vi "AudioTest.SoundCheck Data Log Analysis_Module.vi"(6 "PlotColors":u32[](array[colorbox])=[56063, 16776722, 16730898, 16711925, 6618880], 7 "LimColors":u32[](array[colorbox])=[16448250, 16448250, 16448250, 16448250, 16448250, 16448250], 11 "Module Config":T3={"Name"="AudioGraphs", "Parent Q"=refnum, "Is Child?"=FALSE, "Index"=0, "Dirs"={"Root"=path "", "Config"=path "C:/MTE/Audio Test/Config", "Logs"=path "", "Reports"=path "", "App Data"=path ""}, "Simulate"=FALSE, "SimCtrl"=refnum}) -> ()   [LabVIEW 2018]
uses:
  <vilib>/KATE/Module/Module Config.ctl
  <vilib>/KATE/Queues/Q.Element.ctl
  <vilib>/KATE/Module/Module.Working Dirs.ctl
  Common/Utils/Results/Result.Measurement Item.ctl
  Common/Utils/Results/Result.Measurement and Attribute Item Status.ctl
  TypeDefs/AudioTest.Analysis Data Record.ctl
  TypeDefs/AudioTest.Analysis Folder Navigation Status.ctl
  Common/Utils/Errors/Error.Error Code List.ctl
  <vilib>/KATE/Queues/Queue Utils.lvlib
  <vilib>/KATE/Files/File Utils.lvlib
  <vilib>/KATE/Time/Time Utils.lvlib
  <vilib>/KATE/Module/Module Utils.lvlib
panel:
  in  "Main Tab":enum32{"Graphs", "Results", "Setup"}(tab)
  in  "Graph - Open Composite Sm":bool
  in  "UUT Dir Order":enum16{"Name", "Date"}(ring)
  in  "UUTDir Next":bool
  in  "UUTDir Prev":bool
  in  "Graph - Open Composite":bool
  in  "Go To Results":bool
  in  "Graph Wins - Reset Pos":bool
  in  "Graph Wins - Close":bool
  in  "Graph Wins - Open":bool
  in  "Save to CSV":bool
  in  "X Scale":enum16{"Log", "Linear"}(ring)
  out "Y Units":string
  out "X Units":string
  in  "Next":bool
  in  "Prev":bool
  out "XY Graph":cluster{"X":dbl[], "Y":dbl[]}[](graph)
  in  "Plot":u16(ring)
  in  "SoundCheck Data File":path caption="Data File"
  in  "Load File":bool
  in  "Go To Setup":bool
  in  "Go To Graphs":bool
  out "Meas Data":T1[](array[typedef]) {"Status" items=["LOG", "PASS", "FAIL", "ERROR"]}
  in  "Reinit Config":bool
  out "Graph Cnt":i32
  out "Error":errorcluster
  out "Q Name":string="AudioGraphs"
  in  "Go To Graphs 2":bool
  # "Indiv Graphs"
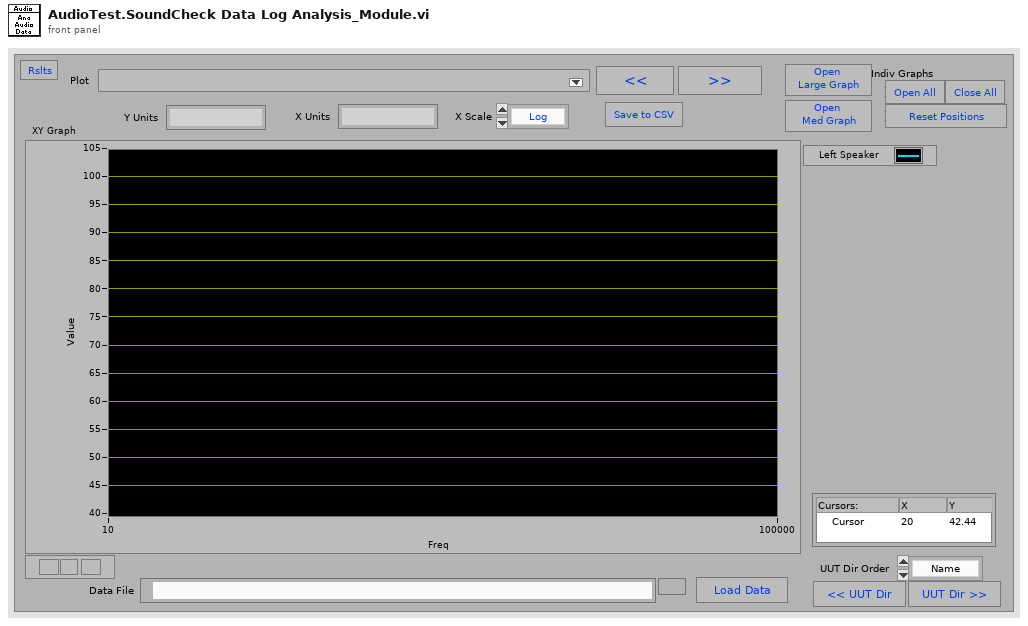
[diagram p1: front panel]
types:
  T1 = typedef "Result.Measurement Item.ctl" = cluster{"Cnt":i32, "Step":string, "Category":string, "Name":string, "Value":string, "Units":string, "LimType":string, "LL":string, "UL":string, "Status":T2, "Code":i32, "Desc":string, "Time":timestamp}
  T2 = typedef "Result.Measurement and Attribute Item Status.ctl" = i32
  T3 = typedef "KATE_Lib.lvlib/Module Utils.lvlib/Module Config.ctl" = cluster{"Name":string, "Parent Q":refnum<queue>, "Is Child?":bool, "Index":i32, "Dirs":T4, "Simulate":bool, "SimCtrl":refnum<vi>}
  T4 = typedef "KATE_Lib.lvlib/Module Utils.lvlib/Module.Working Dirs.ctl" = cluster{"Root":path, "Config":path, "Logs":path, "Reports":path, "App Data":path}
  T5 = typedef "AudioTest.Analysis Data Record.ctl" = cluster{"Name":string, "X Units":string, "Y Units":string, "DataPlots":cluster{"X":dbl[], "Y":dbl[]}[], "LimitPlots":cluster{"X":dbl[], "Y":dbl[]}[], "DataPlotNames":string[], "LimitPlotNames":string[], "Fail":bool}
  T6 = typedef "AudioTest.Analysis Folder Navigation Status.ctl" = cluster{"Index":i32, "Count":i32, "HightEnd":bool, "LowtEnd":bool}
  T7 = enum32{"invalid app kind", "Development System", "Run Time System", "Student Edition", "Embedded LabVIEW", "Evaluation", "Custom"}
  T8 = cluster{"Graphs":T5[], "Config Dir":path, "PlotColors":u32[], "LimColors":u32[], "PlotWins":cluster{"Name":string, "vi ref":refnum<vi>}[], "PlotComp":cluster{"Name":string, "vi ref":refnum<vi>}, "DataFolder":path, "DirNavStatus":T6}
  T9 = typedef "Error.Error Code List.ctl" = i32
  T10 = typedef "KATE_Lib.lvlib/Queue Utils.lvlib/Q.Element.ctl" = cluster{"Cmd":string, "Sub":string, "Data1":variant, "Data2":variant}
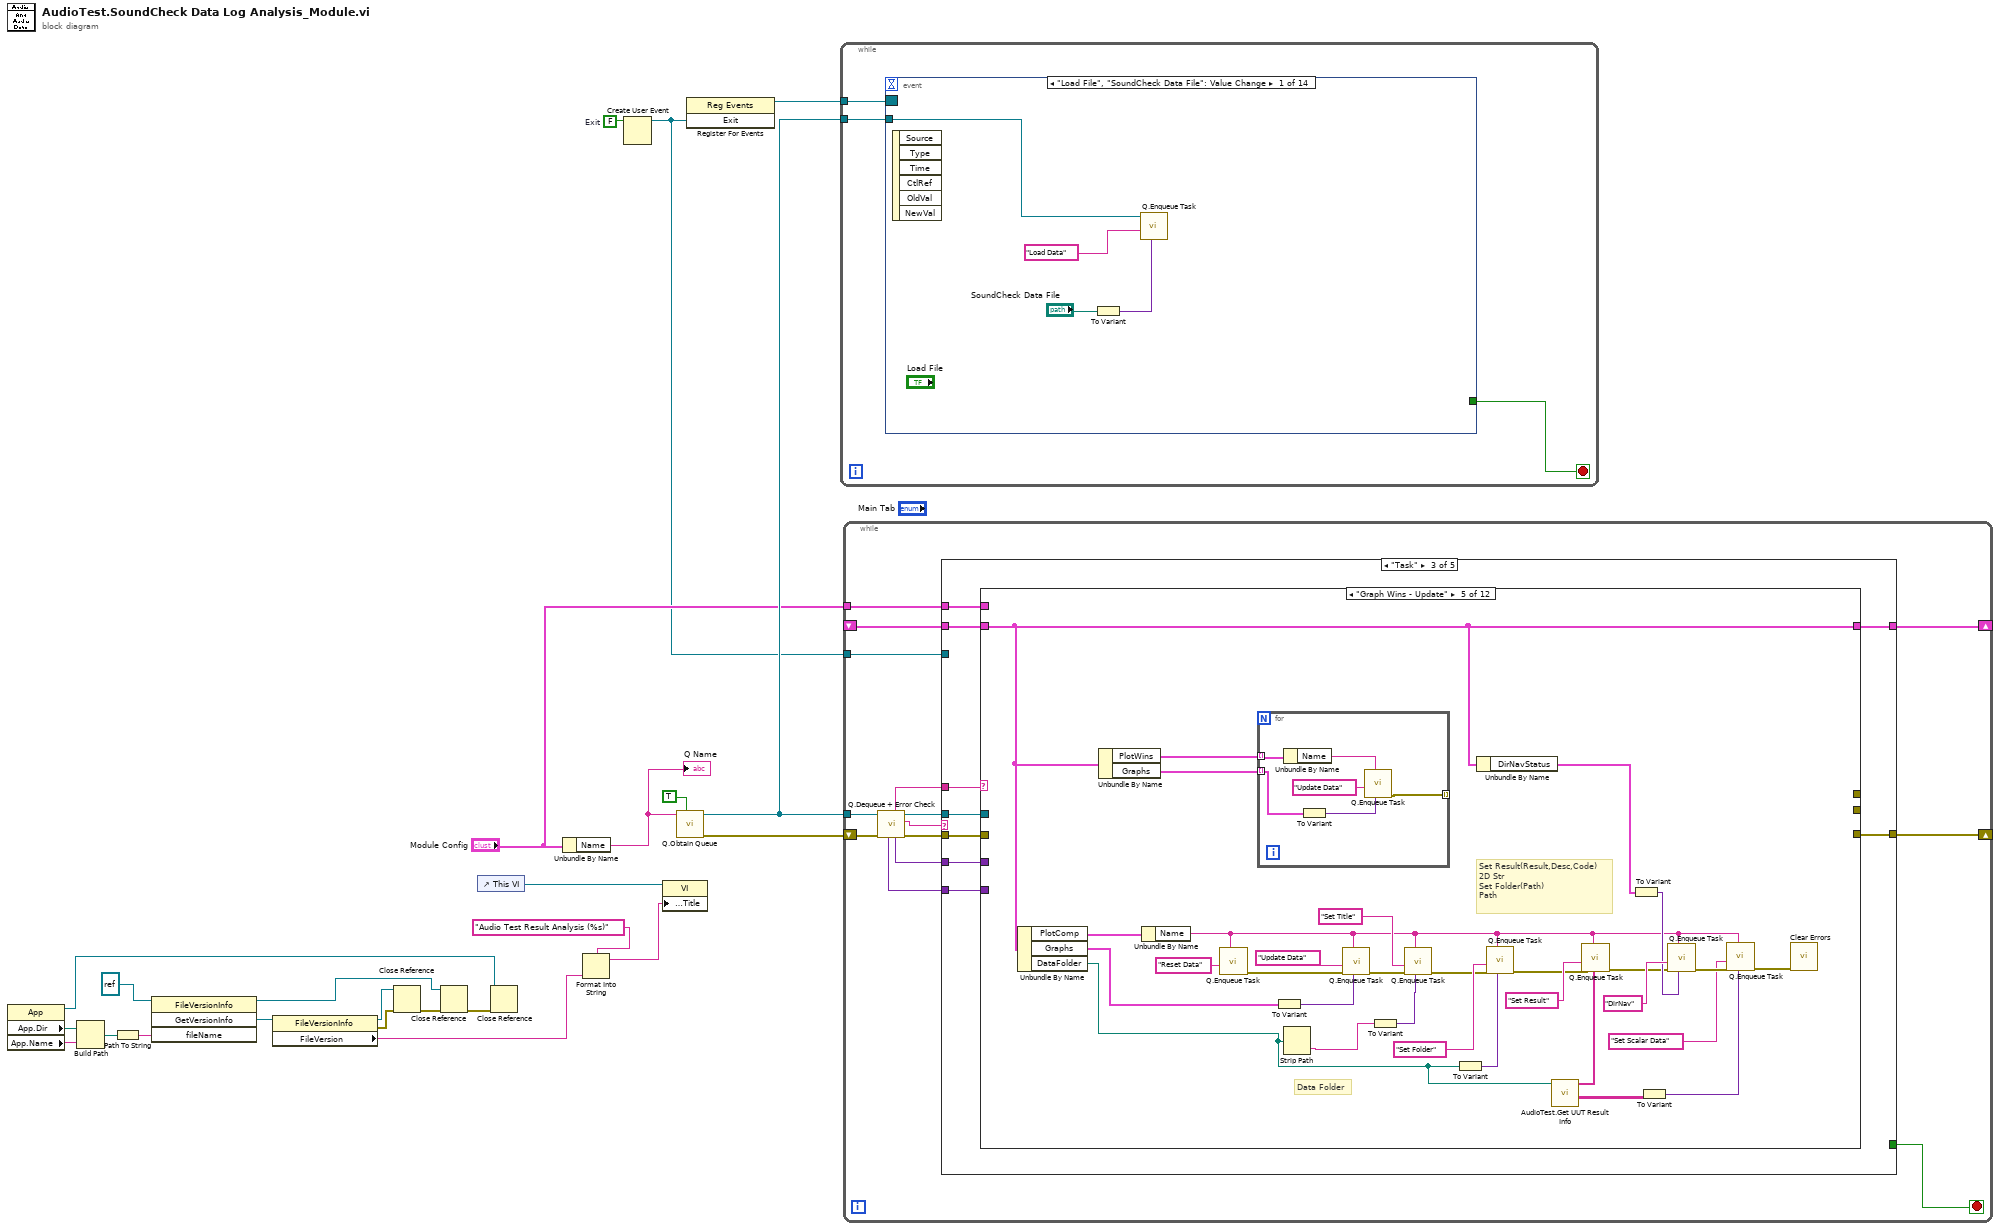
[diagram p0: block diagram]
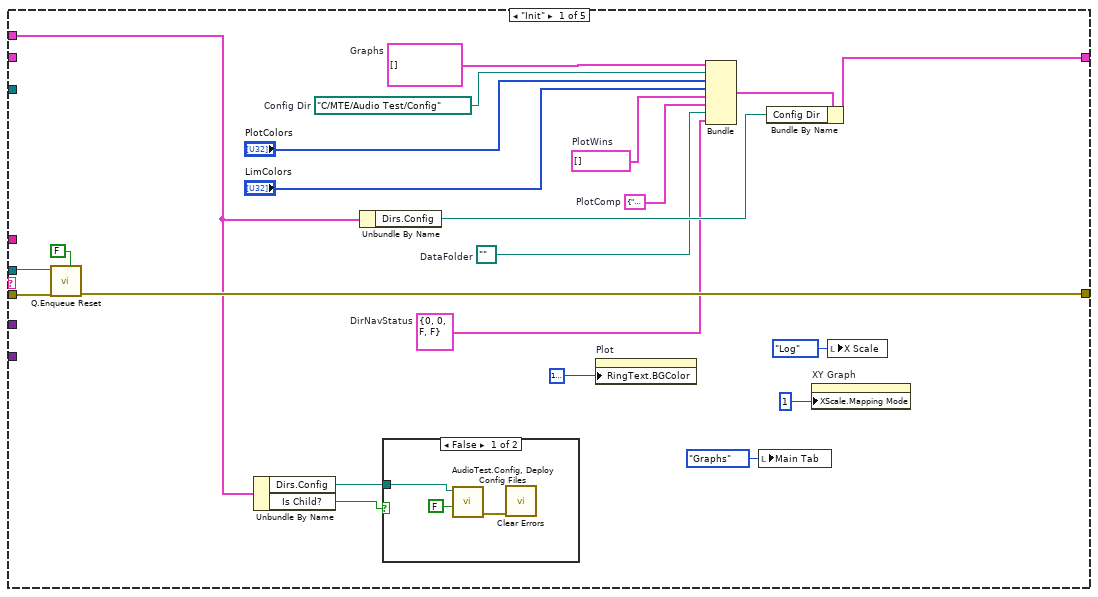
[diagram p2: hidden frame]
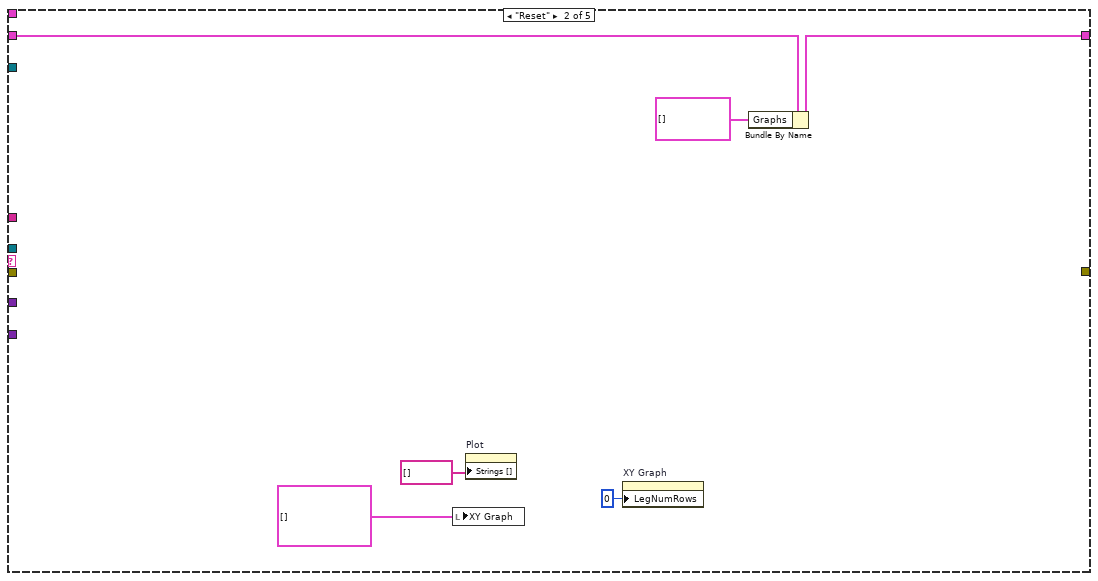
[diagram p4: hidden frame]
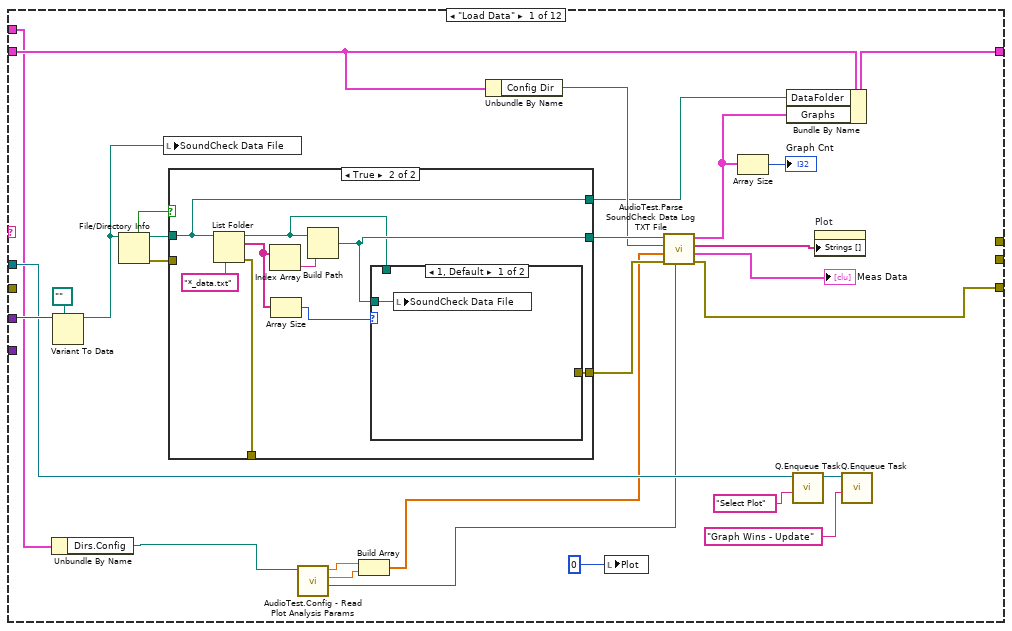
[diagram p5: hidden frame]
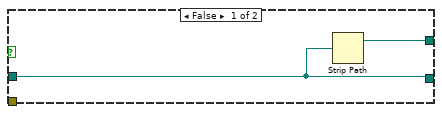
[diagram p6: hidden frame]
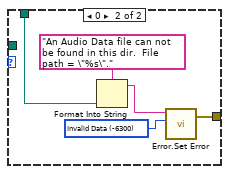
[diagram p7: hidden frame]
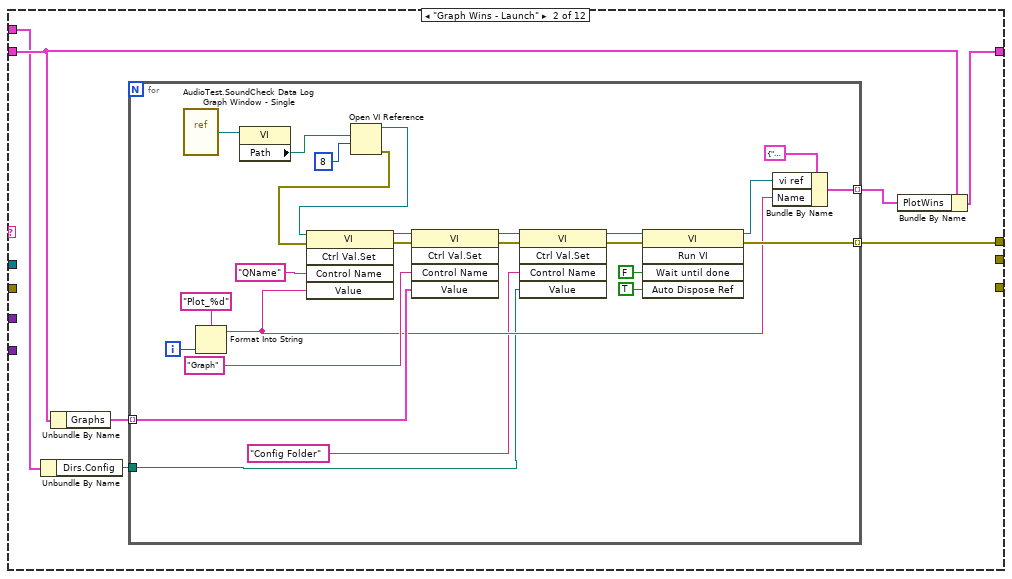
[diagram p8: hidden frame]
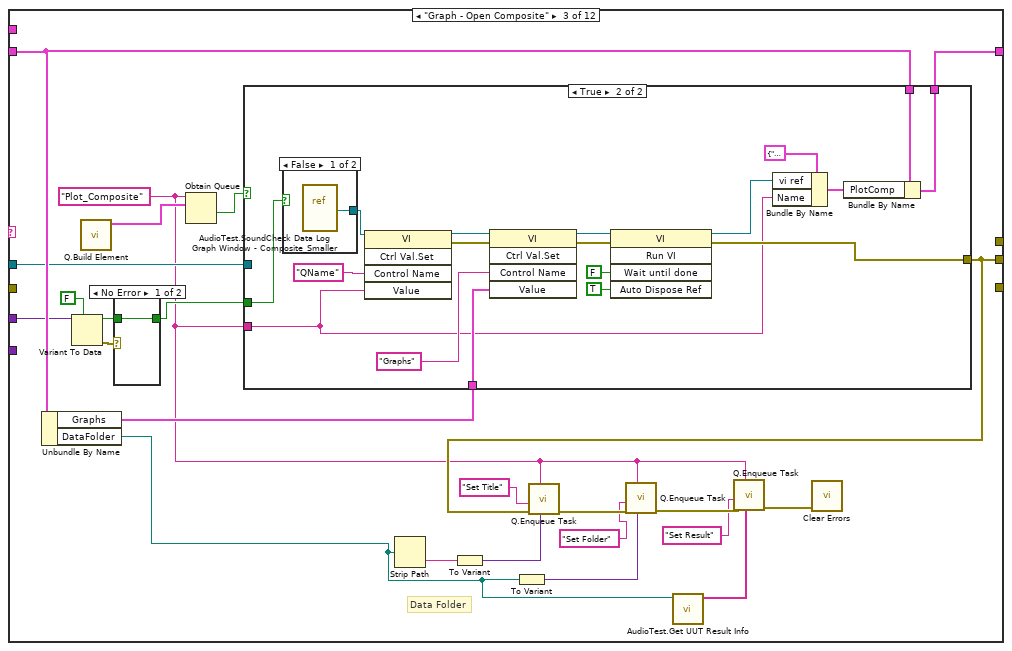
[diagram p9: hidden frame]
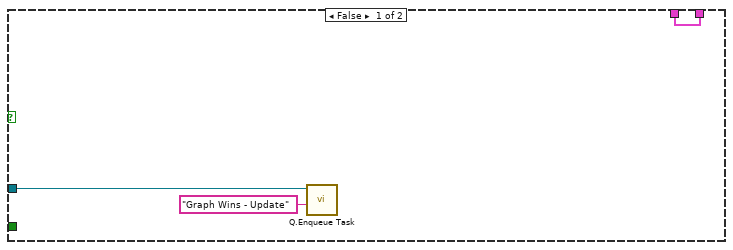
[diagram p11: hidden frame]
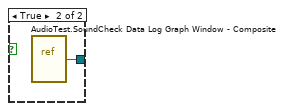
[diagram p12: hidden frame]
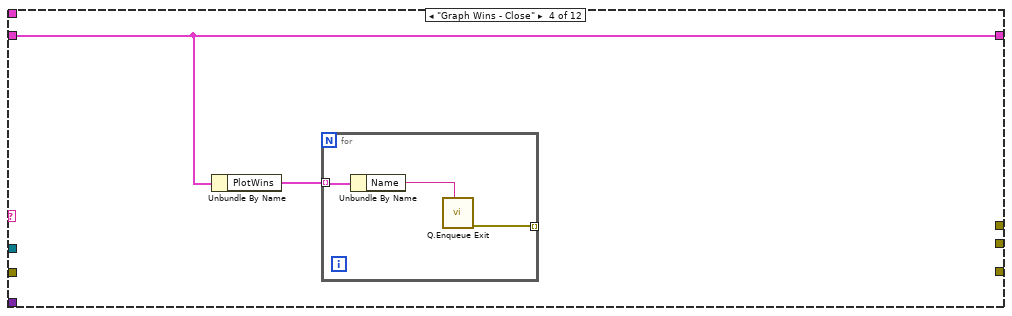
[diagram p13: hidden frame]
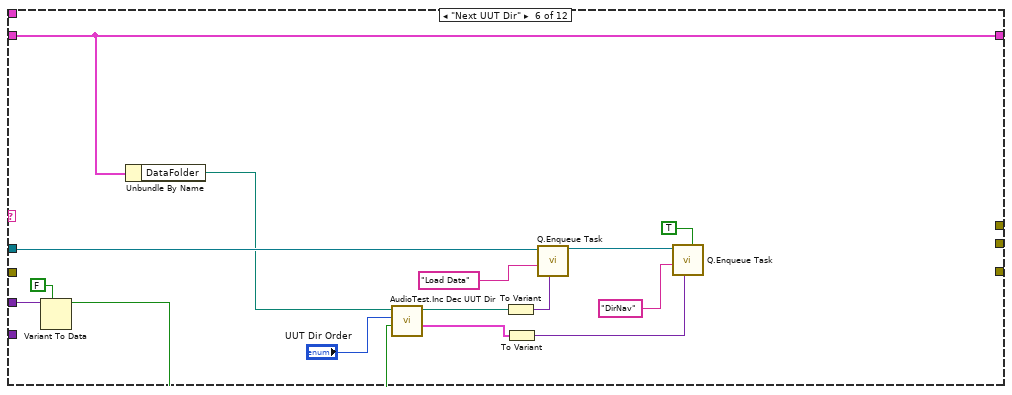
[diagram p14: hidden frame]
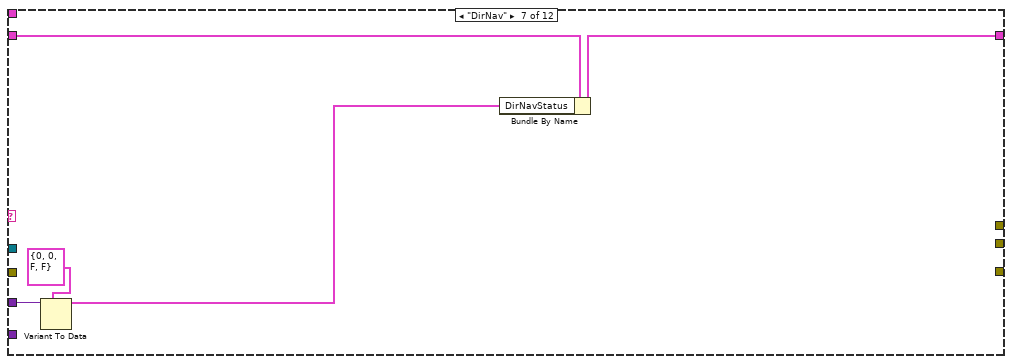
[diagram p15: hidden frame]
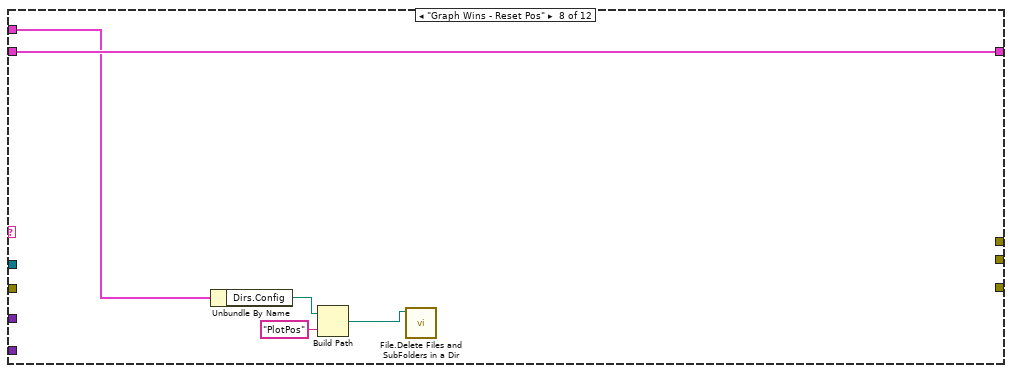
[diagram p16: hidden frame]
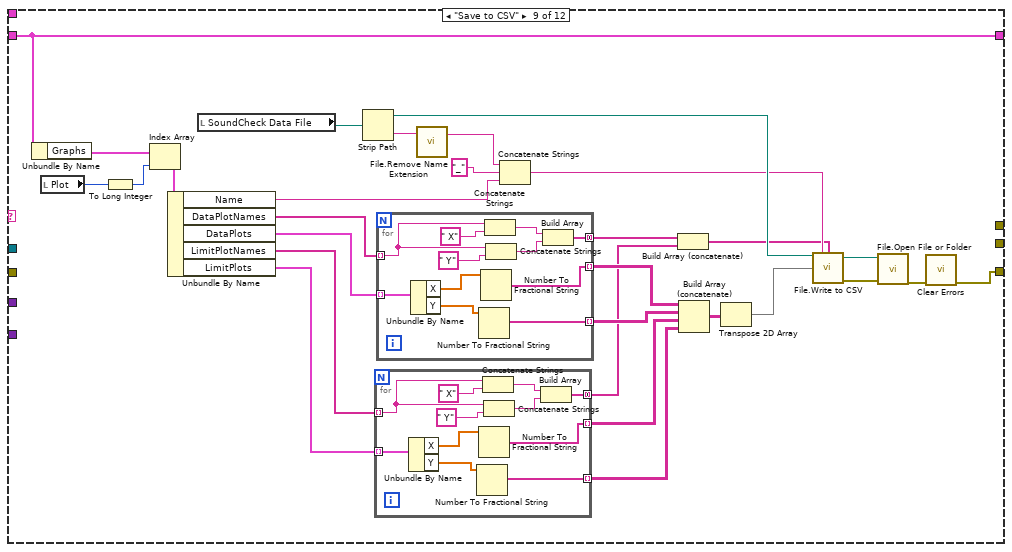
[diagram p17: hidden frame]
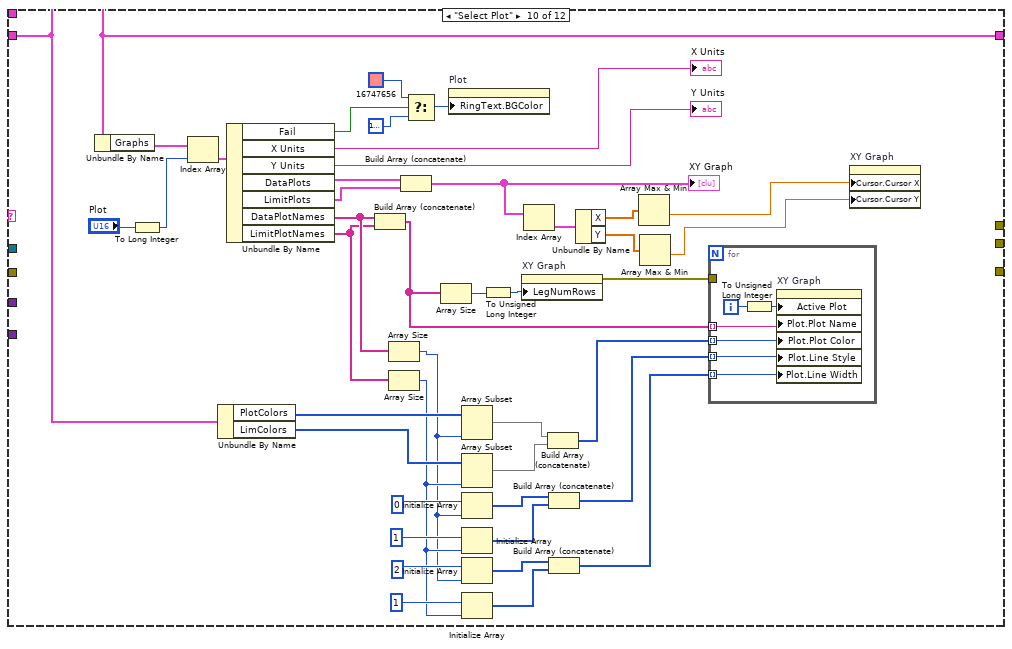
[diagram p18: hidden frame]
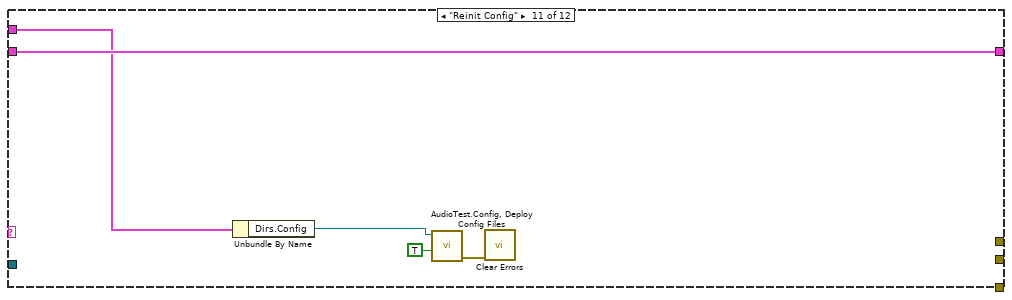
[diagram p19: hidden frame]
diagram:
  w24 = FALSE  # Exit
  n1 = property class="App"() -> (reference out=w3:refnum<vi>, "App.Dir"=w7:path, "App.Name"=w6:string)  [unwired: 2 in, 1 out]
  n2 = Build Path(base path=w7, name or relative path=w6) -> (appended path=w5:path)
  n3 = Path To String(path=w5) -> (string=w13:string)
  n4 = invoke class="FileVersionInfo" method="GetVersionInfo"(reference=refnum<k24> refnum, "fileName"=w13) -> (reference out=w9:refnum<k24>, "GetVersionInfo"=w14:refnum<k24>)  [unwired: 2 in, 2 out]
  n5 = property class="FileVersionInfo"(reference=w14) -> (reference out=w12:refnum<k24>, error out=w11:errorcluster, "FileVersion"=w2:string)  [unwired: 1 in]
  n6 = Close Reference(reference=w12, error in (no error)=w11) -> (error out=w10:errorcluster)
  n7 = Close Reference(reference=w9, error in (no error)=w10) -> (error out=w4:errorcluster)
  n8 = control-ref of="This VI"() -> (w17:refnum<vi>)
  n9 = Close Reference(reference=w3, error in (no error)=w4) -> ()  [unwired: 1 out]
  n10 = Unbundle By Name("Module Config") -> ("Name"=w19:string)
  "Q Name" <- w19
  n11 = Format Into String(format string="Audio Test Result Analysis (%s)", w2) -> (resulting string=w15:string)  [unwired: 2 in, 1 out]
  n12 = Create User Event(user event datatype=w24) -> (user event=w1:refnum<user-event>)  [unwired: 1 in, 1 out]
  n13 = property class="VI"(reference=w17, "Front Panel.Title"=w15) -> ()  [unwired: 1 in, 2 out]
  n14 = call <vilib>:"Q.Obtain Queue.vi"("Enqueue Init"=TRUE, "Q Name"=w19) -> ("error out"=w21:errorcluster, "Q Out"=w20:refnum<queue>)  [unwired: 7 in, 1 out]
  n15 = register-events(w1) -> (reference out=w23:refnum<event-registration>)  [unwired: 2 in, 1 out]
  n16 = while {
    tunnel: w23 -> [w27]
    tunnel: w20 -> [w26]
    stop <- w25 stop-if-true
    n17 = event shown="[0] \"Load File\", \"SoundCheck Data File\": Value Change" {
      selector: w27 -> [_ _ _ _ _ _ _ _ _ _ _ _ _ _]
      dyn-events: _ -> [_ _ _ _ _ _ _ _ _ _ _ _ _ _]
      timeout: _ -> [_ _ _ _ _ _ _ _ _ _ _ _ _ _]
      tunnel: w26 -> [w30 w33 _ w46 w48 w50 w53 w59 w60 w62 _ w75 w89 w92]
      tunnel: [_ _ _ _ _ _ _ _ _ _ _ _ w90 TRUE] -> w25
      event "Load File", "SoundCheck Data File": Value Change {
        n18 = event-data() -> ()  [unwired: 1 in, 6 out]
        n19 = To Variant(anything="SoundCheck Data File") -> (Variant=w28:variant)
        n20 = call <vilib>:"Q.Enqueue Task.vi"("Data1"=w28, "Task Name"="Load Data", "Q In"=w30) -> ()  [unwired: 7 in, 2 out]
      }
      event "UUTDir Prev", "UUTDir Next": Value Change {
        n21 = event-data() -> ()  [unwired: 1 in, 6 out]
        n22 = To Variant(anything="UUTDir Next") -> (Variant=w34:variant)
        n23 = call <vilib>:"Q.Enqueue Task.vi"("Data1"=w34, "Task Name"="Next UUT Dir", "Q In"=w33) -> ()  [unwired: 7 in, 2 out]
      }
      event "Go To Setup", "Go To Results", "Go To Graphs 2", "Go To Graphs": Value Change {
        n24 = event-data() -> ()  [unwired: 1 in, 6 out]
        n25 = Or(x="Go To Graphs 2", y="Go To Graphs") -> (x .or. y?=w37:bool)
        n26 = case shown="False" w37 {
          tunnel: [w42 enum32{"Graphs", "Results", "Setup"}."Graphs" ("Main Tab")] -> w40
          tunnel: "Go To Results" -> [w41 _]
          frame False {
            n27 = case shown="False" w41 {
              tunnel: [enum32{"Graphs", "Results", "Setup"}."Setup" ("Main Tab") enum32{"Graphs", "Results", "Setup"}."Results" ("Main Tab")] -> w42
              frame False {
              }
              frame True {
              }
            }
          }
          frame True {
          }
        }
        n28 = local write "Main Tab"(w40) -> ()
      }
      event "Reinit Config": Value Change {
        n29 = event-data() -> ()  [unwired: 1 in, 6 out]
        n30 = call <vilib>:"Q.Enqueue Task.vi"("Task Name"="Reinit Config", "Q In"=w46) -> ()  [unwired: 8 in, 2 out]
      }
      event "Plot": Value Change {
        n31 = event-data() -> ()  [unwired: 1 in, 6 out]
        n32 = call <vilib>:"Q.Enqueue Task.vi"("Task Name"="Select Plot", "Q In"=w48) -> ()  [unwired: 8 in, 2 out]
      }
      event "Save to CSV": Value Change {
        n33 = event-data() -> ()  [unwired: 1 in, 6 out]
        n34 = call <vilib>:"Q.Enqueue Task.vi"("Task Name"="Save to CSV", "Q In"=w50) -> ()  [unwired: 8 in, 2 out]
      }
      event "Graph Wins - Open": Value Change {
        n35 = event-data() -> ()  [unwired: 1 in, 6 out]
        n36 = call <vilib>:"Q.Enqueue Task.vi"("Task Name"="Graph Wins - Close", "Q In"=w53) -> ("Q Out"=w52:refnum<queue>)  [unwired: 8 in, 1 out]
        n37 = call <vilib>:"Q.Enqueue Task.vi"("Task Name"="Graph Wins - Launch", "Q In"=w52) -> ()  [unwired: 8 in, 2 out]
      }
      event "Graph - Open Composite", "Graph - Open Composite Sm": Value Change {
        n38 = event-data() -> ()  [unwired: 1 in, 6 out]
        n39 = To Variant(anything="Graph - Open Composite") -> (Variant=w57:variant)
        n40 = call <vilib>:"Q.Enqueue Task.vi"("Data1"=w57, "Task Name"="Graph - Open Composite", "Q In"=w59) -> ()  [unwired: 7 in, 2 out]
      }
      event "Graph Wins - Reset Pos": Value Change {
        n41 = event-data() -> ()  [unwired: 1 in, 6 out]
        n42 = call <vilib>:"Q.Enqueue Task.vi"("Task Name"="Graph Wins - Reset Pos", "Q In"=w60) -> ()  [unwired: 8 in, 2 out]
      }
      event "Graph Wins - Close": Value Change {
        n43 = event-data() -> ()  [unwired: 1 in, 6 out]
        n44 = call <vilib>:"Q.Enqueue Task.vi"("Task Name"="Graph Wins - Close", "Q In"=w62) -> ()  [unwired: 8 in, 2 out]
      }
      event "X Scale": Value Change {
        n45 = event-data() -> ()  [unwired: 1 in, 6 out]
        n46 = case shown="\"Log\", Default" "X Scale" {
          tunnel: [u8 1 u8 0] -> w64
          frame "Log", Default {
          }
          frame "Linear" {
          }
        }
        n47 = property on="XY Graph" class="XYGraph (strict)"("XScale.Mapping Mode"=w64) -> ()  [unwired: 2 in, 2 out]
      }
      event "Next", "Prev": Value Change {
        n48 = event-data() -> ()  [unwired: 1 in, 6 out]
        n49 = local read "Graph Cnt"() -> (w71:i32)
        n50 = local read "Plot"() -> (w73:u16)
        n51 = Decrement(x=w71) -> (x-1=w70:i32)
        n52 = To Long Integer(number=w73) -> (32bit integer=w72:i32)
        n53 = case shown="False" "Next" {
          tunnel: w72 -> [w81 w87]
          tunnel: [w77 w85] -> w69
          tunnel: w70 -> [w80 w86]
          frame False {
            n54 = Decrement(x=w81) -> (x-1=w78:i32)
            n55 = Less Than 0?(x=w78) -> (x < 0?=w79:bool)
            n56 = Select(t=w80, s=w79, f=w78) -> (s? t:f=w77:i32)
          }
          frame True {
            n57 = Increment(x=w87) -> (x+1=w82:i32)
            n58 = Greater?(x=w82, y=w86) -> (0:w84:bool)
            n59 = Select(t=0, s=w84, f=w82) -> (s? t:f=w85:i32)
          }
        }
        n60 = To Unsigned Word Integer(number=w69) -> (unsigned 16bit integer=w68:u16)
        n61 = call <vilib>:"Q.Enqueue Task.vi"("Task Name"="Select Plot", "Q In"=w75) -> ()  [unwired: 8 in, 2 out]
        n62 = local write "Plot"(w68) -> ()
      }
      event Panel Close? {
        w90 = TRUE
        n63 = event-data() -> ()  [unwired: 1 in, 4 out]
        n64 = call <vilib>:"Q.Enqueue Exit.vi"("Q In"=w89) -> ("error out"=w88:errorcluster)  [unwired: 9 in, 1 out]
        n65 = call <vilib>:"Clear Errors.vi"("error in (no error)"=w88) -> ()  [unwired: 5 in, 2 out]
        n66 = event-data("Discard?"=w90) -> ()  [unwired: 1 in, 1 out]
      }
      event User Event {
        n67 = event-data() -> ()  [unwired: 1 in, 5 out]
        n68 = call <vilib>:"Q.Enqueue Exit.vi"("Q In"=w92) -> ("error out"=w91:errorcluster)  [unwired: 9 in, 1 out]
        n69 = call <vilib>:"Clear Errors.vi"("error in (no error)"=w91) -> ()  [unwired: 5 in, 2 out]
      }
    }
  }
  n70 = while {
    shift-right: [w99] -> _
    shift-left: w21 -> [w104]
    tunnel: w20 -> [w102]
    shift-right: [w97] -> _
    shift-left: _ -> [w96]
    tunnel: "Module Config" -> [w95]
    tunnel: w1 -> [w94]
    stop <- w98 stop-if-true
    n71 = call <vilib>:"Q.Dequeue + Error Check.vi"("Error In"=w104, "Q In"=w102) -> ("error out"=w105:errorcluster, "Cmd"=w107:string, "Q Out"=w106:refnum<queue>, "Data1"=w101:variant, "Sub"=w103:string, "Data2"=w100:variant)  [unwired: 4 in]
    n72 = case shown="\"Task\"" w107 {
      tunnel: w106 -> [w129 _ w146 w446 _]
      tunnel: w105 -> [w128 _ w145 w445 _]
      tunnel: w103 -> [_ _ w147 _ _]
      tunnel: w101 -> [_ _ w144 _ _]
      tunnel: w100 -> [_ _ w143 _ _]
      tunnel: [w126 _ w140 _ _] -> w99
      tunnel: [_ _ _ _ TRUE] -> w98
      tunnel: [w118 w137 w141 w448 w458] -> w97
      tunnel: w96 -> [_ w136 w142 w448 w458]
      tunnel: w95 -> [w111 _ w139 _ w462]
      tunnel: w94 -> [_ _ _ _ w450]
      frame "Init" {
        w108 = T6 {"Index"=0, "Count"=0, "HightEnd"=FALSE, "LowtEnd"=FALSE}  # DirNavStatus
        w109 = path ""  # DataFolder
        w114 = cluster{"Name":string, "vi ref":refnum<vi>} {"Name"="", "vi ref"=refnum}  # PlotComp
        w116 = cluster{"Name":string, "vi ref":refnum<vi>}[] []  # PlotWins
        w122 = path "C:/MTE/Audio Test/Config"  # Config Dir
        w125 = T5[] []  # Graphs
        n73 = call <vilib>:"Q.Enqueue Reset.vi"("Top of Q(T)"=FALSE, "Error In"=w128, "Q In"=w129) -> ("error out"=w126:errorcluster)  [unwired: 7 in, 1 out]
        n74 = Unbundle By Name(w111) -> ("Dirs.Config"=w112:path, "Is Child?"=w110:bool)
        n75 = Unbundle By Name(w111) -> ("Dirs.Config"=w117:path)
        n76 = case shown="False" w110 {
          tunnel: w112 -> [w131 _]
          frame False {
            n77 = call "AudioTest.Config, Deploy Config Files.vi"("SkipIfExists(F)/Overwrite(T)"=FALSE, "Config Folder"=w131) -> ("error out"=w132:errorcluster)  [unwired: 9 in]
            n78 = call <vilib>:"Clear Errors.vi"("error in (no error)"=w132) -> ()  [unwired: 5 in, 2 out]
          }
          frame True {
          }
        }
        n79 = property on="Plot" class="Ring (strict)"("RingText.BGColor"=u32 16777216 ("Color Box")) -> ()  [unwired: 2 in, 2 out]
        n80 = Bundle("Graphs"=w125, "Config Dir"=w122, "PlotColors"="PlotColors", "LimColors"="LimColors", "PlotWins"=w116, "PlotComp"=w114, "DataFolder"=w109, "DirNavStatus"=w108) -> (w119:T8)  [unwired: 1 in]
        n81 = local write "Main Tab"(enum32{"Graphs", "Results", "Setup"}."Graphs" ("Main Tab")) -> ()
        n82 = Bundle By Name(cluster=w119, "Config Dir"=w117) -> (w118:T8)
        n83 = property on="XY Graph" class="XYGraph (strict)"("XScale.Mapping Mode"=u8 1) -> ()  [unwired: 2 in, 2 out]
        n84 = local write "X Scale"(enum16{"Log", "Linear"}."Log" ("X Scale")) -> ()
      }
      frame "Reset" {
        n85 = local write "XY Graph"(cluster{"X":dbl[], "Y":dbl[]}[] [] ("appended array")) -> ()
        n86 = property on="Plot" class="Ring (strict)"("Strings []"=string[] []) -> ()  [unwired: 2 in, 2 out]
        n87 = property on="XY Graph" class="XYGraph (strict)"("LegNumRows"=u32 0 ("Legend:Number of Rows")) -> ()  [unwired: 2 in, 2 out]
        n88 = Bundle By Name(cluster=w136, "Graphs"=T5[] []) -> (w137:T8)
      }
      frame "Task" {
        n89 = case shown="\"Graph Wins - Update\"" w147 {
          tunnel: w146 -> [w166 _ w238 _ _ w324 _ _ _ _ _ _]
          tunnel: w145 -> [_ _ _ _ _ _ _ _ _ _ _ _]
          tunnel: w144 -> [w169 _ w243 _ _ w323 w333 _ _ _ _ _]
          tunnel: w143 -> [_ _ _ _ _ _ _ _ _ _ _ _]
          tunnel: w142 -> [w162 w198 w246 w274 w286 w320 w330 w338 w363 w419 w442 w443]
          tunnel: [w167 w197 w245 w274 w286 w320 w331 w338 w363 w419 w442 w443] -> w141
          tunnel: [w165 _ _ _ _ _ _ _ w340 _ _ _] -> w140
          tunnel: [_ w195 _ _ _ _ _ _ _ _ _ _] -> _
          tunnel: w139 -> [w155 w194 _ _ _ _ _ w337 _ _ w440 _]
          tunnel: [_ _ w227 _ _ _ _ _ _ _ _ _] -> _
          frame "Load Data" {
            n90 = Unbundle By Name(w155) -> ("Dirs.Config"=w154:path)
            n91 = Variant To Data(type=path "", Variant=w169) -> (data=w164:path)  [unwired: 1 in, 1 out]
            n92 = File/Directory Info(path=w164) -> (path out=w171:path, directory=w172:bool, error out=w174:errorcluster)  [unwired: 1 in, 4 out]
            n93 = local write "SoundCheck Data File"(w164) -> ()
            n94 = case shown="True" w172 {
              tunnel: w171 -> [w177 w178]
              tunnel: [w177 w185] -> w173
              tunnel: w174 -> [_ _]
              tunnel: [_ w184] -> _
              tunnel: [_ w180] -> w175
              tunnel: [w176 w178] -> w148
              frame False {
                n95 = Strip Path(path=w177) -> (stripped path=w176:path)  [unwired: 1 out]
              }
              frame True {
                n96 = List Folder(path=w178, pattern="*_data.txt") -> (path out=w179:path, filenames=w183:string[], error out=w184:errorcluster)  [unwired: 2 in, 1 out]
                n97 = Index Array(array=w183) -> (element=w181:string)  [unwired: 1 in]
                n98 = Array Size(array=w183) -> (size(s)=w182:i32)
                n99 = Build Path(base path=w179, name or relative path=w181) -> (appended path=w185:path)
                n100 = case shown="1, Default" w182 {
                  tunnel: w185 -> [w187 _]
                  tunnel: [_ w189] -> w180
                  tunnel: w179 -> [_ w188]
                  frame 1, Default {
                    n101 = local write "SoundCheck Data File"(w187) -> ()
                  }
                  frame 0 {
                    w190 = T9 -6300 items=["No Error"=0, "Abort"=-2, "Misc"=-5000, "Fixture Error"=-5100, "File IO - General"=-5200, "FIle IO - Config Error"=-5201, "Instrument - General"=-5300, "Instrument - Serial Com"=-5301, "Instrument - Camera"=-5302, "Instrument - PS"=-5303, "Instrument - Oscilloscope"=-5304, "Instrument - Function Gen"=-5305, "Instrument - Load"=-5306, "Instrument - Meter"=-5307, "Instrument - Power Control"=-5308, "Instrument - Motion"=-5309, "Instrument - RF"=-5310, "System Exe"=-5400, "Image Processing"=-5500, "Communication"=-5600, "Script - Syntax Error"=-6000, "Script - Invalid Name or Param"=-6100, "Script - Timeout"=-6200, "Invalid Data"=-6300, "FW Update Error"=-6500] ("Std Code")
                    n102 = Format Into String(format string="An Audio Data file can not be found in this dir.  File path = \"%s\"." ("Desc"), w188) -> (resulting string=w192:string)  [unwired: 2 in, 1 out]
                    n103 = call "Error.Set Error.vi"("Code"=w190, "Desc"=w192) -> ("error out"=w189:errorcluster)  [unwired: 5 in]
                  }
                }
              }
            }
            n104 = call "AudioTest.Config - Read Plot Analysis Params.vi"("Config Dir"=w154) -> ("Avg(F)/Float(T)"=w152:bool, "End Freq"=w156:dbl, "Start Freq"=w157:dbl)  [unwired: 8 in]
            n105 = Build Array(w157, w156) -> (w153:dbl[])
            n106 = Unbundle By Name(w162) -> ("Config Dir"=w161:path)
            n107 = local write "Plot"(0) -> ()
            n108 = call "AudioTest.Parse SoundCheck Data Log TXT File.vi"("Lim Center at Average(f), Float at center"=w152, "error in"=w175, "Start_End"=w153, "Config Folder"=w161, "SoundCheck Data File"=w173) -> ("error out"=w165:errorcluster, "Meas Rslt"=→"Meas Data":T1[], "Graph Names"=w163:string[], "Graphs"=w160:T5[])  [unwired: 3 in]
            n109 = Array Size(array=w160) -> (size(s)=→"Graph Cnt":i32)
            n110 = Bundle By Name(cluster=w162, "DataFolder"=w148, "Graphs"=w160) -> (w167:T8)
            n111 = call <vilib>:"Q.Enqueue Task.vi"("Task Name"="Select Plot", "Q In"=w166) -> ("Q Out"=w150:refnum<queue>)  [unwired: 8 in, 1 out]
            n112 = property on="Plot" class="Ring (strict)"("Strings []"=w163) -> ()  [unwired: 2 in, 2 out]
            n113 = call <vilib>:"Q.Enqueue Task.vi"("Task Name"="Graph Wins - Update", "Q In"=w150) -> ()  [unwired: 8 in, 2 out]
          }
          frame "Graph Wins - Launch" {
            n114 = Unbundle By Name(w194) -> ("Dirs.Config"=w193:path)
            n115 = Unbundle By Name(w198) -> ("Graphs"=w199:T5[])
            n116 = for {
              tunnel: w199 -> [w216] mode=indexing
              tunnel: [w215] -> w195 mode=indexing
              tunnel: [w211] -> w196 mode=indexing
              tunnel: w193 -> [w200]
              i -> [w217]
              n117 = vi-ref "AudioTest.SoundCheck Data Log Graph Window - Single.vi"() -> (w210:refnum<vi>)
              n118 = Format Into String(format string="Plot_%d", w217) -> (resulting string=w213:string)  [unwired: 2 in, 1 out]
              n119 = property class="VI"(reference=w210) -> ("Path"=w209:path)  [unwired: 1 in, 2 out]
              n120 = Open VI Reference(vi path=w209, options=8) -> (vi reference=w208:refnum<vi>, error out=w206:errorcluster)  [unwired: 4 in]
              n121 = invoke class="VI" method="Ctrl Val.Set"(reference=w208, error in=w206, "Control Name"="QName", "Value"=w213) -> (reference out=w222:refnum<vi>, error out=w221:errorcluster)  [unwired: 1 in, 3 out]
              n122 = invoke class="VI" method="Ctrl Val.Set"(reference=w222, error in=w221, "Control Name"="Graph", "Value"=w216) -> (reference out=w205:refnum<vi>, error out=w204:errorcluster)  [unwired: 1 in, 3 out]
              n123 = invoke class="VI" method="Ctrl Val.Set"(reference=w205, error in=w204, "Control Name"="Config Folder", "Value"=w200) -> (reference out=w202:refnum<vi>, error out=w203:errorcluster)  [unwired: 1 in, 3 out]
              n124 = invoke class="VI" method="Run VI"(reference=w202, error in=w203, "Wait until done"=FALSE ("Wait Until Done"), "Auto Dispose Ref"=TRUE ("Auto Dispose Reference")) -> (reference out=w212:refnum<vi>, error out=w215:errorcluster)  [unwired: 1 in, 3 out]
              n125 = Bundle By Name(cluster=cluster{"Name":string, "vi ref":refnum<vi>} {"Name"="", "vi ref"=refnum} ("Service"), "vi ref"=w212, "Name"=w213) -> (w211:cluster{"Name":string, "vi ref":refnum<vi>})
            }
            n126 = Bundle By Name(cluster=w198, "PlotWins"=w196) -> (w197:T8)
          }
          frame "Graph - Open Composite" {
            w226 = "Plot_Composite"
            # "Data Folder"
            n127 = Unbundle By Name(w246) -> ("Graphs"=w248:T5[], "DataFolder"=w225:path)
            n128 = Variant To Data(type=FALSE, Variant=w243) -> (data=w240:bool, error out=w241:errorcluster)  [unwired: 1 in]
            n129 = call <vilib>:"Q.Build Element.vi"() -> ("Q.Element"=w244:T10)  [unwired: 11 in]
            n130 = case shown="No Error" w241 {
              tunnel: w240 -> [w249 _]
              tunnel: [w249 _] -> w239
              frame No Error {
              }
              frame Error {
              }
            }
            n131 = Obtain Queue(name (unnamed)=w226, element data type=w244) -> (created new?=w247:bool)  [unwired: 3 in, 2 out]
            n132 = case shown="True" w247 {
              tunnel: w248 -> [_ w270]
              tunnel: [_ w258] -> w227
              tunnel: w226 -> [_ w257]
              tunnel: w246 -> [w252 w255]
              tunnel: [w252 w254] -> w245
              tunnel: w238 -> [w251 _]
              tunnel: w239 -> [_ w253]
              frame False {
                n133 = call <vilib>:"Q.Enqueue Task.vi"("Task Name"="Graph Wins - Update", "Q In"=w251) -> ()  [unwired: 8 in, 2 out]
              }
              frame True {
                n134 = case shown="False" w253 {
                  tunnel: [w271 w272] -> w259
                  frame False {
                    n135 = vi-ref "AudioTest.SoundCheck Data Log Graph Window - Composite_Smaller.vi"() -> (w271:refnum<vi>)
                  }
                  frame True {
                    n136 = vi-ref "AudioTest.SoundCheck Data Log Graph Window - Composite.vi"() -> (w272:refnum<vi>)
                  }
                }
                n137 = invoke class="VI" method="Ctrl Val.Set"(reference=w259, "Control Name"="QName", "Value"=w257) -> (reference out=w267:refnum<vi>, error out=w266:errorcluster)  [unwired: 2 in, 3 out]
                n138 = invoke class="VI" method="Ctrl Val.Set"(reference=w267, error in=w266, "Control Name"="Graphs", "Value"=w270) -> (reference out=w261:refnum<vi>, error out=w260:errorcluster)  [unwired: 1 in, 3 out]
                n139 = invoke class="VI" method="Run VI"(reference=w261, error in=w260, "Wait until done"=FALSE ("Wait Until Done"), "Auto Dispose Ref"=TRUE ("Auto Dispose Reference")) -> (reference out=w262:refnum<vi>, error out=w258:errorcluster)  [unwired: 1 in, 3 out]
                n140 = Bundle By Name(cluster=cluster{"Name":string, "vi ref":refnum<vi>} {"Name"="", "vi ref"=refnum} ("Service"), "vi ref"=w262, "Name"=w257) -> (w256:cluster{"Name":string, "vi ref":refnum<vi>})
                n141 = Bundle By Name(cluster=w255, "PlotComp"=w256) -> (w254:T8)
              }
            }
            n142 = Strip Path(path=w225) -> (name=w236:string)  [unwired: 1 out]
            n143 = To Variant(anything=w236) -> (Variant=w237:variant)
            n144 = To Variant(anything=w225) -> (Variant=w235:variant)
            n145 = call <vilib>:"Q.Enqueue Task.vi"("Data1"=w237, "Q Name"=w226, "Error In"=w227, "Task Name"="Set Title") -> ("error out"=w234:errorcluster)  [unwired: 6 in, 1 out]
            n146 = call <vilib>:"Q.Enqueue Task.vi"("Data1"=w235, "Q Name"=w226, "Error In"=w234, "Task Name"="Set Folder") -> ("error out"=w233:errorcluster)  [unwired: 6 in, 1 out]
            n147 = call "AudioTest.Get UUT Result Info.vi"("Folder"=w225) -> ("Result"=w231:string[])  [unwired: 9 in, 1 out]
            n148 = call <vilib>:"Q.Enqueue Task.vi"("Data1"=w231, "Q Name"=w226, "Error In"=w233, "Task Name"="Set Result") -> ("error out"=w232:errorcluster)  [unwired: 6 in, 1 out]
            n149 = call <vilib>:"Clear Errors.vi"("error in (no error)"=w232) -> ()  [unwired: 5 in, 2 out]
          }
          frame "Graph Wins - Close" {
            n150 = Unbundle By Name(w274) -> ("PlotWins"=w273:cluster{"Name":string, "vi ref":refnum<vi>}[])
            n151 = for {
              tunnel: w273 -> [w277] mode=indexing
              tunnel: [w275] -> _ mode=indexing
              n152 = Unbundle By Name(w277) -> ("Name"=w276:string)
              n153 = call <vilib>:"Q.Enqueue Exit.vi"("Q Name"=w276) -> ("error out"=w275:errorcluster)  [unwired: 9 in, 1 out]
            }
          }
          frame "Graph Wins - Update" {
            # "Set Result(Result,Desc,Code)\n2D Str\nSet Folder(Path)\nPath"
            # "Data Folder"
            n154 = Unbundle By Name(w286) -> ("PlotComp"=w303:cluster{"Name":string, "vi ref":refnum<vi>}, "Graphs"=w302:T5[], "DataFolder"=w289:path)
            n155 = Unbundle By Name(w286) -> ("PlotWins"=w307:cluster{"Name":string, "vi ref":refnum<vi>}[], "Graphs"=w306:T5[])
            n156 = Unbundle By Name(w303) -> ("Name"=w284:string)
            n157 = call <vilib>:"Q.Enqueue Task.vi"("Q Name"=w284, "Task Name"="Reset Data") -> ("error out"=w290:errorcluster)  [unwired: 8 in, 1 out]
            n158 = for {
              tunnel: w307 -> [w313] mode=indexing
              tunnel: [w309] -> _ mode=indexing
              tunnel: w306 -> [w312] mode=indexing
              n159 = Unbundle By Name(w313) -> ("Name"=w310:string)
              n160 = To Variant(anything=w312) -> (Variant=w311:variant)
              n161 = call <vilib>:"Q.Enqueue Task.vi"("Data1"=w311, "Q Name"=w310, "Task Name"="Update Data") -> ("error out"=w309:errorcluster)  [unwired: 7 in, 1 out]
            }
            n162 = To Variant(anything=w302) -> (Variant=w304:variant)
            n163 = Strip Path(path=w289) -> (name=w299:string)  [unwired: 1 out]
            n164 = call <vilib>:"Q.Enqueue Task.vi"("Data1"=w304, "Q Name"=w284, "Error In"=w290, "Task Name"="Update Data") -> ("error out"=w298:errorcluster)  [unwired: 6 in, 1 out]
            n165 = To Variant(anything=w299) -> (Variant=w301:variant)
            n166 = call <vilib>:"Q.Enqueue Task.vi"("Data1"=w301, "Q Name"=w284, "Error In"=w298, "Task Name"="Set Title") -> ("error out"=w294:errorcluster)  [unwired: 6 in, 1 out]
            n167 = To Variant(anything=w289) -> (Variant=w296:variant)
            n168 = Unbundle By Name(w286) -> ("DirNavStatus"=w285:T6)
            n169 = call <vilib>:"Q.Enqueue Task.vi"("Data1"=w296, "Q Name"=w284, "Error In"=w294, "Task Name"="Set Folder") -> ("error out"=w293:errorcluster)  [unwired: 6 in, 1 out]
            n170 = call "AudioTest.Get UUT Result Info.vi"("Folder"=w289) -> ("Misc Data"=w279:string[][], "Result"=w292:string[])  [unwired: 9 in]
            n171 = call <vilib>:"Q.Enqueue Task.vi"("Data1"=w292, "Q Name"=w284, "Error In"=w293, "Task Name"="Set Result") -> ("error out"=w283:errorcluster)  [unwired: 6 in, 1 out]
            n172 = To Variant(anything=w285) -> (Variant=w287:variant)
            n173 = To Variant(anything=w279) -> (Variant=w280:variant)
            n174 = call <vilib>:"Q.Enqueue Task.vi"("Data1"=w287, "Q Name"=w284, "Error In"=w283, "Task Name"="DirNav") -> ("error out"=w282:errorcluster)  [unwired: 6 in, 1 out]
            n175 = call <vilib>:"Q.Enqueue Task.vi"("Data1"=w280, "Q Name"=w284, "Error In"=w282, "Task Name"="Set Scalar Data") -> ("error out"=w281:errorcluster)  [unwired: 6 in, 1 out]
            n176 = call <vilib>:"Clear Errors.vi"("error in (no error)"=w281) -> ()  [unwired: 5 in, 2 out]
          }
          frame "Next UUT Dir" {
            n177 = Variant To Data(type=FALSE, Variant=w323) -> (data=w321:bool)  [unwired: 1 in, 1 out]
            n178 = Unbundle By Name(w320) -> ("DataFolder"=w319:path)
            n179 = call "AudioTest.Inc Dec UUT Dir.vi"("Increment"=w321, "UUT Dir Order"="UUT Dir Order", "SoundCheck Data File"=w319) -> ("FolderNavStatus"=w316:T6, "Next Folder"=w326:path)  [unwired: 7 in]
            n180 = To Variant(anything=w326) -> (Variant=w328:variant)
            n181 = To Variant(anything=w316) -> (Variant=w315:variant)
            n182 = call <vilib>:"Q.Enqueue Task.vi"("Data1"=w328, "Task Name"="Load Data", "Q In"=w324) -> ("Q Out"=w318:refnum<queue>)  [unwired: 7 in, 1 out]
            n183 = call <vilib>:"Q.Enqueue Task.vi"("Top of Q"=TRUE, "Data1"=w315, "Task Name"="DirNav", "Q In"=w318) -> ()  [unwired: 6 in, 2 out]
          }
          frame "DirNav" {
            n184 = Variant To Data(type=T6 {"Index"=0, "Count"=0, "HightEnd"=FALSE, "LowtEnd"=FALSE} ("FolderNavStatus"), Variant=w333) -> (data=w329:T6)  [unwired: 1 in, 1 out]
            n185 = Bundle By Name(cluster=w330, "DirNavStatus"=w329) -> (w331:T8)
          }
          frame "Graph Wins - Reset Pos" {
            n186 = Unbundle By Name(w337) -> ("Dirs.Config"=w335:path)
            n187 = Build Path(base path=w335, name or relative path="PlotPos") -> (appended path=w334:path)
            n188 = call <vilib>:"File.Delete Files and SubFolders in a Dir.vi"("Dir"=w334) -> ()  [unwired: 9 in, 2 out]
          }
          frame "Save to CSV" {
            n189 = Unbundle By Name(w363) -> ("Graphs"=w367:T5[])
            n190 = local read "Plot"() -> (w366:u16)
            n191 = To Long Integer(number=w366) -> (32bit integer=w365:i32)
            n192 = Index Array(array=w367, index=w365) -> (element=w364:T5)
            n193 = Unbundle By Name(w364) -> ("Name"=w358:string, "DataPlotNames"=w356:string[], "DataPlots"=w357:cluster{"X":dbl[], "Y":dbl[]}[], "LimitPlotNames"=w349:string[], "LimitPlots"=w348:cluster{"X":dbl[], "Y":dbl[]}[])
            n194 = local read "SoundCheck Data File"() -> (w362:path)
            n195 = Strip Path(path=w362) -> (stripped path=w353:path, name=w361:string)
            n196 = for {
              tunnel: w348 -> [w378] mode=indexing
              tunnel: w349 -> [w374] mode=indexing
              tunnel: [w372] -> w347 mode=indexing
              tunnel: [w371] -> w346 mode=indexing
              tunnel: [w368] -> w345 mode=concatenating
              n197 = Unbundle By Name(w378) -> ("X"=w377:dbl[], "Y"=w376:dbl[])
              n198 = Number To Fractional String(number=w376) -> (F-format string=w371:string[])  [unwired: 3 in]
              n199 = Number To Fractional String(number=w377) -> (F-format string=w372:string[])  [unwired: 3 in]
              n200 = Concatenate Strings(w374, " X" ("string")) -> (w370:string)
              n201 = Concatenate Strings(w374, " Y" ("string")) -> (w369:string)
              n202 = Build Array(w370, w369) -> (w368:string[])
            }
            n203 = for {
              tunnel: w357 -> [w389] mode=indexing
              tunnel: w356 -> [w385] mode=indexing
              tunnel: [w383] -> w355 mode=indexing
              tunnel: [w382] -> w354 mode=indexing
              tunnel: [w379] -> w350 mode=concatenating
              n204 = Unbundle By Name(w389) -> ("X"=w388:dbl[], "Y"=w387:dbl[])
              n205 = Number To Fractional String(number=w387) -> (F-format string=w382:string[])  [unwired: 3 in]
              n206 = Number To Fractional String(number=w388) -> (F-format string=w383:string[])  [unwired: 3 in]
              n207 = Concatenate Strings(w385, " X" ("string")) -> (w381:string)
              n208 = Concatenate Strings(w385, " Y" ("string")) -> (w380:string)
              n209 = Build Array(w381, w380) -> (w379:string[])
            }
            n210 = call <vilib>:"File.Remove Name Extension.vi"("File Name"=w361) -> ("Name Less Ext"=w359:string)  [unwired: 1 in, 1 out]
            n211 = Concatenate Strings(w359, "_", w358) -> (w352:string)
            n212 = Build Array (concatenate)(w350, w345) -> (w344:string[])
            n213 = Build Array (concatenate)(w355, w354, w347, w346) -> (w343:string[][])
            n214 = Transpose 2D Array(2D array=w343) -> (transposed array=w351:string[][])
            n215 = call <vilib>:"File.Write to CSV.vi"("Folder"=w353, "FileRootName"=w352, "Header"=w344, "2D"=w351) -> ("File Path"=w342:path, "error out"=w341:errorcluster)  [unwired: 10 in]
            n216 = call <vilib>:"File.Open File or Folder.vi"("Error In"=w341, "Path"=w342) -> ("Error Out"=w339:errorcluster)  [unwired: 9 in]
            n217 = call <vilib>:"Clear Errors.vi"("error in (no error)"=w339) -> ("error out"=w340:errorcluster)  [unwired: 5 in, 1 out]
          }
          frame "Select Plot" {
            n218 = Unbundle By Name(w419) -> ("Graphs"=w426:T5[])
            n219 = To Long Integer(number="Plot") -> (32bit integer=w429:i32)
            n220 = Index Array(array=w426, index=w429) -> (element=w427:T5)
            n221 = Unbundle By Name(w419) -> ("PlotColors"=w416:u32[], "LimColors"=w415:u32[])
            n222 = Unbundle By Name(w427) -> ("Fail"=w396:bool, "X Units"=→"X Units":string, "Y Units"=→"Y Units":string, "DataPlots"=w425:cluster{"X":dbl[], "Y":dbl[]}[], "LimitPlots"=w424:cluster{"X":dbl[], "Y":dbl[]}[], "DataPlotNames"=w418:string[], "LimitPlotNames"=w417:string[])
            n223 = Build Array (concatenate)(w418, w417) -> (w420:string[])
            n224 = Array Size(array=w418) -> (size(s)=w401:i32)
            n225 = Array Size(array=w417) -> (size(s)=w402:i32)
            n226 = Build Array (concatenate)(w425, w424) -> (w395:cluster{"X":dbl[], "Y":dbl[]}[])
            "XY Graph" <- w395
            n227 = Select(t=u32 16747656 ("Color Box"), s=w396, f=u32 16777216 ("Color Box")) -> (s? t:f=w398:u32)
            n228 = Array Size(array=w420) -> (size(s)=w423:i32)
            n229 = property on="Plot" class="Ring (strict)"("RingText.BGColor"=w398) -> ()  [unwired: 2 in, 2 out]
            n230 = Array Subset(array=w416, length=w401) -> (w414:u32[])  [unwired: 1 in]
            n231 = Array Subset(array=w415, length=w402) -> (w413:u32[])  [unwired: 1 in]
            n232 = Initialize Array(u8 0 ("Plot.Line Style"), w401) -> (w409:u8[])
            n233 = Initialize Array(u8 1 ("Plot.Line Style"), w402) -> (w408:u8[])
            n234 = Initialize Array(u8 2 ("Plot.Line Style"), w401) -> (w405:u8[])
            n235 = Initialize Array(u8 1 ("Plot.Line Style"), w402) -> (w406:u8[])
            n236 = To Unsigned Long Integer(number=w423) -> (unsigned 32bit integer=w422:u32)
            n237 = property on="XY Graph" class="XYGraph (strict)"("LegNumRows"=w422) -> (error out=w421:errorcluster)  [unwired: 2 in, 1 out]
            n238 = Index Array(array=w395) -> (element=w394:cluster{"X":dbl[], "Y":dbl[]})  [unwired: 1 in]
            n239 = Build Array (concatenate)(w414, w413) -> (w412:u32[])
            n240 = Build Array (concatenate)(w409, w408) -> (w407:u8[])
            n241 = Build Array (concatenate)(w405, w406) -> (w400:u8[])
            n242 = Unbundle By Name(w394) -> ("X"=w393:dbl[], "Y"=w392:dbl[])
            n243 = Array Max & Min(array=w393) -> (min value=w391:dbl)  [unwired: 3 out]
            n244 = Array Max & Min(array=w392) -> (min value=w390:dbl)  [unwired: 3 out]
            n245 = for {
              tunnel: w420 -> [w435] mode=indexing
              tunnel: w421 -> [_]
              tunnel: w412 -> [w434] mode=indexing
              tunnel: w407 -> [w433] mode=indexing
              tunnel: w400 -> [w432] mode=indexing
              i -> [w436]
              n246 = To Unsigned Long Integer(number=w436) -> (unsigned 32bit integer=w437:u32)
              n247 = property on="XY Graph" class="XYGraph (strict)"("Active Plot"=w437, "Plot.Plot Name"=w435, "Plot.Plot Color"=w434, "Plot.Line Style"=w433, "Plot.Line Width"=w432) -> ()  [unwired: 2 in, 2 out]
            }
            n248 = property on="XY Graph" class="XYGraph (strict)"("Cursor.Cursor X"=w391, "Cursor.Cursor Y"=w390) -> ()  [unwired: 2 in, 2 out]
          }
          frame "Reinit Config" {
            n249 = Unbundle By Name(w440) -> ("Dirs.Config"=w441:path)
            n250 = call "AudioTest.Config, Deploy Config Files.vi"("SkipIfExists(F)/Overwrite(T)"=TRUE, "Config Folder"=w441) -> ("error out"=w439:errorcluster)  [unwired: 9 in]
            n251 = call <vilib>:"Clear Errors.vi"("error in (no error)"=w439) -> ()  [unwired: 5 in, 2 out]
          }
          frame Default {
          }
        }
      }
      frame "Error", Default {
        # "Do Nothing (for now)"
        n252 = call <vilib>:"Q.Enqueue Reset.vi"("Top of Q(T)"=FALSE, "Error In"=w445, "Q In"=w446) -> ("error out"=w444:errorcluster)  [unwired: 7 in, 1 out]
        n253 = call <vilib>:"Clear Errors.vi"("error in (no error)"=w444) -> ()  [unwired: 5 in, 2 out]
        "Error" <- w445
      }
      frame "Exit" {
        n254 = Generate User Event(user event=w450, event data cluster=TRUE ("event data")) -> ()  [unwired: 2 in, 2 out]
        n255 = Unbundle By Name(w462) -> ("Is Child?"=w461:bool)
        n256 = property class="App"() -> ("App.Kind"=w466:T7)  [unwired: 2 in, 2 out]
        n257 = Not(x=w461) -> (.not. x?=w460:bool)
        n258 = Unbundle By Name(w458) -> ("PlotWins"=w459:cluster{"Name":string, "vi ref":refnum<vi>}[], "PlotComp"=w454:cluster{"Name":string, "vi ref":refnum<vi>})
        n259 = Equal?(x=w466, y=T7."Run Time System" ("Application:Kind")) -> (x = y?=w464:bool)
        n260 = And(x=w460, y=w464) -> (x .and. y?=w463:bool)
        n261 = for {
          tunnel: w459 -> [w469] mode=indexing
          tunnel: [w468] -> w453
          n262 = Unbundle By Name(w469) -> ("Name"=w470:string)
          n263 = call <vilib>:"Q.Enqueue Exit.vi"("Q Name"=w470) -> ("error out"=w468:errorcluster)  [unwired: 9 in, 1 out]
        }
        n264 = Unbundle By Name(w454) -> ("Name"=w455:string)
        n265 = call <vilib>:"Q.Enqueue Exit.vi"("Q Name"=w455) -> ("error out"=w451:errorcluster)  [unwired: 9 in, 1 out]
        n266 = Merge Errors(w453, w451) -> (w452:errorcluster)
        n267 = call <vilib>:"Time.Inline Delay.vi"("error in (no error)"=w452, "Wait(ms)"=u32 50) -> ("error out"=w457:errorcluster)  [unwired: 8 in, 1 out]
        n268 = case shown="True" w463 {
          selector: w463 -> [_ w471]
          tunnel: w457 -> [_ _]
          frame False {
          }
          frame True {
            n269 = Quit LabVIEW(quit? (T)=w471) -> ()
          }
        }
      }
    }
  }
